vi "SGDA-Stop.vi"(0 "Wait for DAQ to stop? (T)":bool=TRUE, 7 "Clear ActiveX (F)":bool, 11 "error in (no error)":errorcluster) -> (15 "error out":errorcluster)   [LabVIEW 2020]
doc: "Sets global variables that terminate the main DAQ loop."
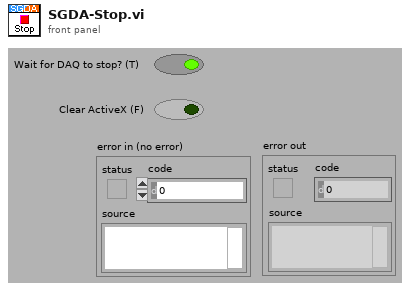
[diagram p1: front panel]
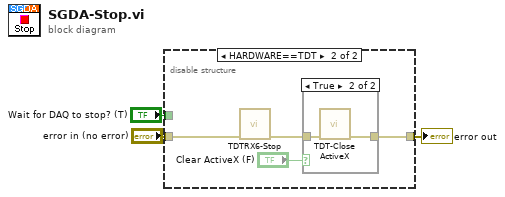
[diagram p0: block diagram]
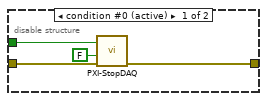
[diagram p2: hidden frame]
diagram:
  n1 = disable-structure shown="HARDWARE==TDT" {
    disable-tunnel: "error in (no error)" -> [w7 w11]
    disable-tunnel: [w6 w9] -> w2
    disable-tunnel: "Wait for DAQ to stop? (T)" -> [w4 _]
    frame condition #0 (active) {
      n2 = call "PXI-StopDAQ.vi"("error in (no error)"=w7, "Reset (T)"=FALSE, "Wait for DAQ to stop? (T)"=w4) -> ("error out"=w6:errorcluster)  [unwired: 4 in]
    }
    frame condition #1 {
      n3 = call "TDTRX6-Stop.vi"("error in (no error)"=w11) -> ("error out"=w10:errorcluster)  [unwired: 14 in]
      n4 = case shown="True" "Clear ActiveX (F)" {
        tunnel: w10 -> [w12 w14]
        tunnel: [w12 w13] -> w9
        frame False {
        }
        frame True {
          n5 = call "TDT-Close ActiveX.vi"("error in (no error)"=w14) -> ("error out"=w13:errorcluster)  [unwired: 14 in]
        }
      }
    }
  }
  "error out" <- w2
